vi "State History.vi"(7 "history length (100)":i32=100, 11 "Current State":string) -> (3 "History":string)   [LabVIEW 2019, in "Generator.lvclass"]
uses:
  Generator.lvclass
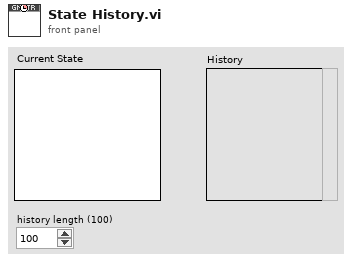
[diagram p1: front panel]
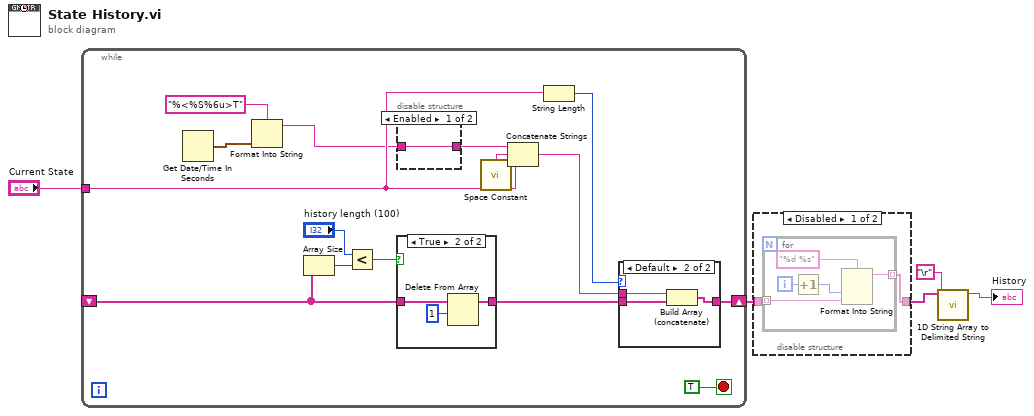
[diagram p0: block diagram]
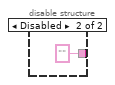
[diagram p3: hidden frame]
diagram:
  n1 = while {
    tunnel: "Current State" -> [w16]
    shift-right: [w17] -> w1
    shift-left: _ -> [w10]
    stop <- TRUE stop-if-true
    n2 = Get Date/Time In Seconds() -> (seconds since 1Jan1904=w8:timestamp)
    n3 = Format Into String(format string="%<%S%6u>T", w8) -> (resulting string=w6:string)  [unwired: 2 in, 1 out]
    n4 = Array Size(array=w10) -> (size(s)=w19:i32)
    n5 = Less?(x="history length (100)", y=w19) -> (x < y?=w13:bool)
    n6 = case shown="True" w13 {
      tunnel: w10 -> [w27 w28]
      tunnel: [w27 w29] -> w20
      frame False {
      }
      frame True {
        n7 = Delete From Array(array=w28, length=1) -> (array with subset deleted=w29:string[])  [unwired: 1 in, 1 out]
      }
    }
    n8 = disable-structure shown="Enabled" {
      disable-tunnel: [w21 "" ("Spinner Out")] -> w15
      disable-tunnel: w6 -> [w21 _]
      frame Enabled {
      }
      frame Disabled {
      }
    }
    n9 = call <vilib>:"Space Constant.vi"() -> ("String"=w14:string)
    n10 = Concatenate Strings(w15, w14, w16) -> (w12:string)
    n11 = String Length(string=w16) -> (length=w11:i32)
    n12 = case shown="Default" w11 {
      tunnel: w20 -> [w23 w25]
      tunnel: [w23 w26] -> w17
      tunnel: w12 -> [_ w24]
      frame 0 {
      }
      frame Default {
        n13 = Build Array (concatenate)(w24, w25) -> (w26:string[])
      }
    }
  }
  n14 = disable-structure shown="Disabled" {
    disable-tunnel: [w32 w38] -> w2
    disable-tunnel: w1 -> [w31 w38]
    frame Disabled {
      n15 = for {
        tunnel: w31 -> [w35] mode=indexing
        tunnel: [w34] -> w32 mode=indexing
        i -> [w36]
        n16 = Increment(x=w36) -> (x+1=w33:i32)
        n17 = Format Into String(format string="%d %s", w33, w35) -> (resulting string=w34:string)  [unwired: 2 in, 1 out]
      }
    }
    frame Enabled {
    }
  }
  n18 = call <vilib>:"1D String Array to Delimited String.vi"("delimiter"="\r", "string array"=w2) -> ("delimited string"=→"History":string)  [unwired: 9 in]
